vi "Mapping References FGV.vi"(7 "Method":enum16{"Get", "Set"}(ring), 8 "Error In":errorcluster, 11 "Map References":T1) -> (0 "Error Out":errorcluster, 3 "Map References Out":T1)   [LabVIEW 2014]
uses:
  Controls/Mapping References.ctl
  C:/Robotic Systems/Products/Surveyor/Software/Ground Station/Data/Mapping DLL/GMap.NET.WindowsForms.dll
  Data/Mapping DLL/GMap.NET.WindowsForms.dll
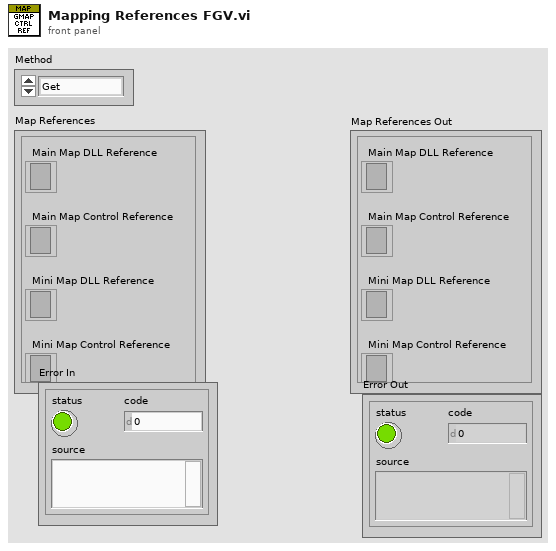
[diagram p1: front panel]
types:
  T1 = typedef "Mapping References.ctl" = cluster{"Main Map DLL Reference":refnum<k24>, "Main Map Control Reference":refnum<k24>, "Mini Map DLL Reference":refnum<k24>, "Mini Map Control Reference":refnum<k24>}
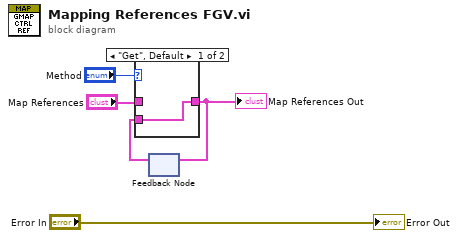
[diagram p0: block diagram]
diagram:
  n1 = feedback #1() -> (w4:T1)  [unwired: 1 in]
  n2 = case shown="\"Get\", Default" "Method" {
    tunnel: "Map References" -> [_ w7]
    tunnel: [w6 w7] -> w3
    tunnel: w4 -> [w6 _]
    frame "Get", Default {
    }
    frame "Set" {
    }
  }
  "Map References Out" <- w3
  n3 = feedback-in #1(w3) -> ()
  "Error Out" <- "Error In"
